vi "Coord window-Trace motor coord.vi"(11 "Coordinates":cluster{"X":sgl, "Y":sgl, "Z":sgl}) -> ()   [LabVIEW 2020]
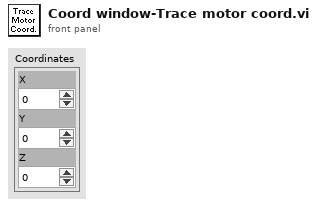
[diagram p1: front panel]
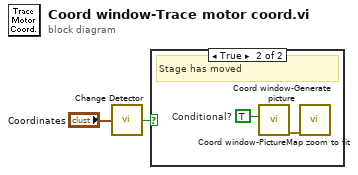
[diagram p0: block diagram]
diagram:
  n1 = call <userlib>:"Change Detector.vi"("Value"="Coordinates") -> ("Changed?"=w2:bool)
  n2 = case shown="True" w2 {
    frame False {
      # "No movement"
    }
    frame True {
      w3 = TRUE  # Conditional?
      # "Stage has moved"
      n3 = call "Coord window-PictureMap zoom to fit.vi"("Conditional?"=w3) -> ("error out"=w4:errorcluster)  [unwired: 10 in]
      n4 = call "Coord window-Generate picture.vi"("error in (no error)"=w4) -> ()  [unwired: 10 in, 1 out]
    }
  }
